vi "Initialize AI Channels.vi"(8 "error in (no error)":errorcluster, 11 "Instrument.Lockin":refnum<class "Instrument.Lockin.lvclass">) -> (0 "error out":errorcluster, 2 "AI Channels":T1[](array[typedef]) {"References" items=["", "1", "2", "3"]}, 3 "Instrument.Lockin out":refnum<class "Instrument.Lockin.lvclass">)   [LabVIEW 2016, in "Instrument.Lockin.lvclass"]
uses:
  Instrument.Lockin.lvclass
  Instrument.Lockinl.UI/Typedefs/AI Channel--Cluster.ctl
  Instrument.Lockin.lvclass/Instrument.Lockin.ctl
  Instrument.Lockinl.UI/Instrument.Lockin.UI.lvclass
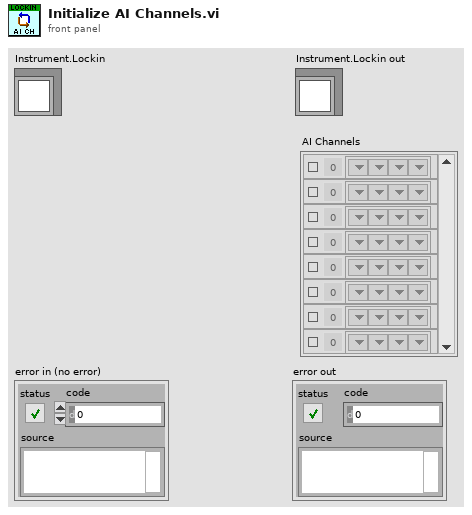
[diagram p1: front panel]
types:
  T1 = typedef "Instrument.Lockin.UI.lvclass/AI Channel--Cluster.ctl" = cluster{"Enable?":bool, "Channel":i32, "References":u16[]}
  T2 = typedef "Lockin.DAQ.lvclass/AI-cluster.ctl" = T1[]
  T3 = typedef "Lockin.DAQ.lvclass/AI.config-array.ctl" = T4[]
  T4 = typedef "Lockin.DAQ.lvclass/AI.config-cluster.ctl" = cluster{"AI.channels":tag, "AI.Coupling":T5, "AI.Range":T6, "input terminal configuration":i32, "DAQ Type":T7}
  T5 = typedef "Lockin.DAQ.lvclass/AI.coupling-enum.ctl" = u16
  T6 = typedef "Lockin.DAQ.lvclass/446xAI-enum.ctl" = enum16{"±0.316", "±1.00", "±3.16", "±10.0", "±31.6", "±42.4"}
  T7 = typedef "Lockin.DAQ.lvclass/DAQType-enum.ctl" = enum16{"None", "USB 4431", "PXI 446x"}
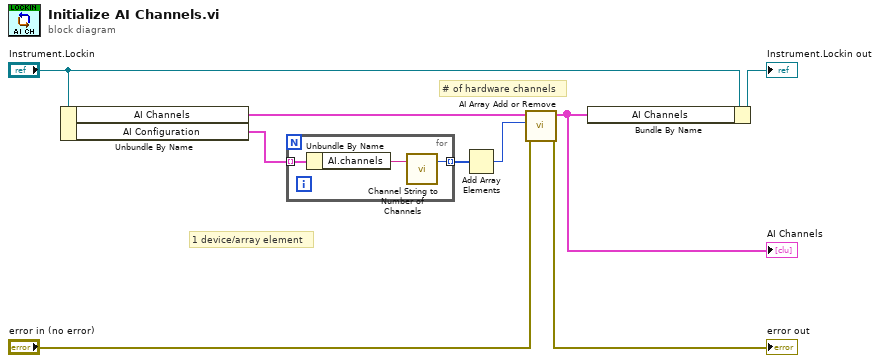
[diagram p0: block diagram]
diagram:
  # "1 device/array element"
  # "# of hardware channels"
  n1 = Unbundle By Name("Instrument.Lockin") -> ("AI Channels"=w3:T2, "AI Configuration"=w2:T3)
  n2 = for {
    tunnel: w2 -> [w12] mode=indexing
    tunnel: [w11] -> w9 mode=indexing
    n3 = Unbundle By Name(w12) -> ("AI.channels"=w10:tag)
    n4 = call "Channel String to Number of Channels.vi"("Channels String"=w10) -> ("# channels"=w11:i32)  [unwired: 2 in]
  }
  n5 = Add Array Elements(numeric array=w9) -> (sum=w1:i32)
  n6 = call "AI Array Add or Remove.vi"("error in (no error)"="error in (no error)", "Size"=w1, "AI Channels"=w3) -> ("error out"=→"error out":errorcluster, "AI Channels out"=w6:T1[])  [unwired: 7 in]
  "AI Channels" <- w6
  n7 = Bundle By Name(cluster="Instrument.Lockin", "AI Channels"=w6) -> (→"Instrument.Lockin out":refnum<class "Instrument.Lockin.lvclass">)
